vi "Generate Report.vi"(8 "error in (no error)":errorcluster, 11 "Text Reports in":refnum<class "Text Reports.lvclass">) -> (0 "error out":errorcluster, 3 "Text Reports out":refnum<class "Text Reports.lvclass">)   [LabVIEW 2020, in "Text Reports.lvclass"]
uses:
  Text Reports.lvclass
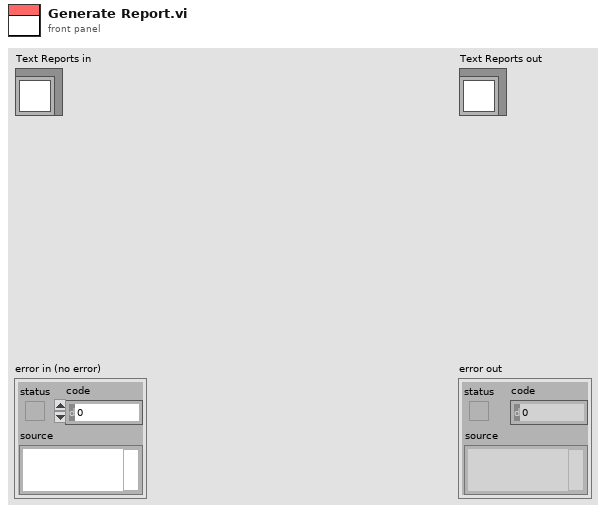
[diagram p1: front panel]
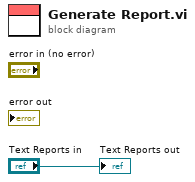
[diagram p0: block diagram]
diagram:
  "Text Reports out" <- "Text Reports in"
